vi "Recrystallise.vi"(8 "error in (no error)":errorcluster, 11 "XAOMsetting":refnum<vi>) -> (0 "error out":errorcluster)   [LabVIEW 2019]
uses:
  controls/xAOMSettings/XAOMsetting.xctl
  controls/GlobalExp.vi
  <vilib>/Utility/error.llb/Error Cluster From Error Code.vi
  <vilib>/rvi/errors/niLvFpgaAdjustHostInterfaceError.vi
  <vilib>/rvi/interface/nirviReadWriteControl/nirviReadWriteControl.xnode
  NiFpgaLv.dll
  <vilib>/rvi/interface/Simulation/niFpgaSimulationCallBeginRW.vi
  Global.lvlib
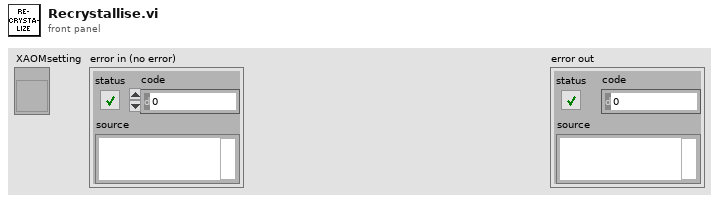
[diagram p1: front panel]
types:
  T1 = cluster{"HighPowerNum":dbl, "LowPowerNum":dbl, "PIDnum":dbl, "DeltaFreq":dbl, "BaseFreq":dbl, "AOMout":dbl, "ButtonSelected":enum16{"PID", "Low", "High"}, "AO3":bool}
  T2 = typedef "MasterExpControl.ctl" = cluster{"Main Steps":dbl, "Main Runs":dbl, "ExpStatus":enum16{"Innit", "Stop", "Idle", "MainRunning", "AuxRunning"}, "Main Current Step":dbl, "ExpNum":dbl, "NewData":bool, "date":string, "command":string, "Stop":bool, "Pause":bool, "Mathematica":string, "Main/Meta":bool, "UpdateMath":bool, "Camera":bool, "MetaExpOver":bool, "NextMetaExp":bool}
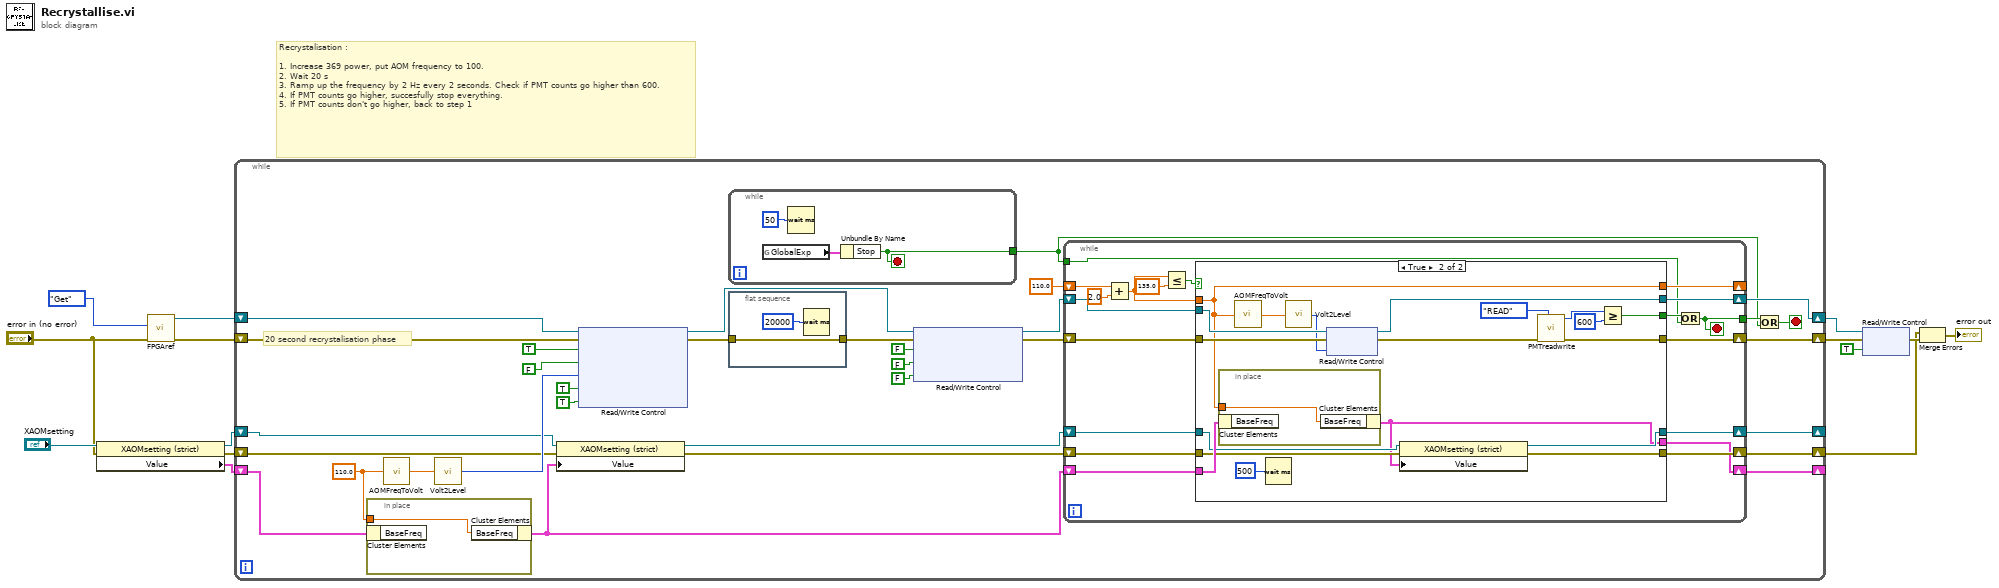
[diagram p0: block diagram]
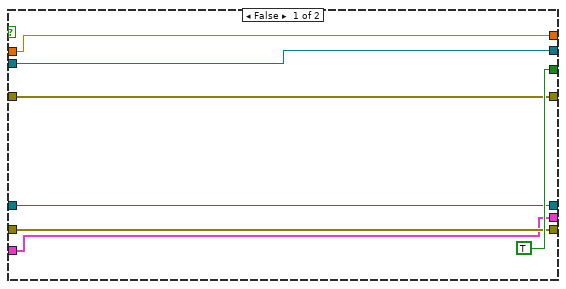
[diagram p2: hidden frame]
diagram:
  # "Recrystalisation :\n\n1. Increase 369 power, put AOM frequency to 100.\n2. Wait 20 s\n3. Ramp up the frequency by 2 Hz every 2 seconds. Check if PMT counts go higher than 600.\n4. If PMT counts go higher, succesfully stop everything.\n5. If PMT counts don't go higher, back to step 1"
  n1 = property class="XAOMsetting (strict)"(reference="XAOMsetting", error in="error in (no error)") -> (reference out=w9:refnum<vi>, error out=w7:errorcluster, "Value"=w8:T1)
  n2 = call "FPGAref.vi"("error in"="error in (no error)", "Enum"=enum16{"Set", "Get"}."Get") -> ("error out"=w5:errorcluster, "FPGA VI Reference Out 2"=w13:refnum<k20>)  [unwired: 4 in]
  n3 = while {
    shift-right: [w30] -> w12
    shift-left: w13 -> [w46]
    shift-right: [w22] -> _
    shift-left: w9 -> [w27]
    shift-right: [w20] -> _
    shift-left: w8 -> [w29]
    shift-right: [w21] -> w2
    shift-left: w7 -> [w26]
    shift-right: [w18] -> w4
    shift-left: w5 -> [w19]
    stop <- w17 stop-if-true
    w28 = 110.0 ("AOM freq")
    # "20 second recrystalisation phase"
    n4 = in-place {
      in-place-border: w28 -> [w50]
      n5 = in-place-cluster #1(w29) -> ()  [unwired: 1 out]
      n6 = in-place-cluster #1("BaseFreq"=w50) -> (w23:T1)
    }
    n7 = call "AOMFreqToVolt.vi"("AOM freq"=w28) -> ("AOM voltage"=w42:dbl)
    n8 = call "Volt2Level.vi"("voltage /V"=w42) -> ("level"=w43:i16)
    n9 = property class="XAOMsetting (strict)"(reference=w27, error in=w26, "Value"=w23) -> (reference out=w25:refnum<vi>, error out=w24:errorcluster)
    n10 = xnode "Read/Write Control"("FPGA VI Reference In"=w46, "error in"=w19, "AO4"=TRUE, "AO3"=FALSE, "AO3 off"=w43, "High power"=TRUE, "override noise eater?"=TRUE) -> ("FPGA VI Reference Out"=w40:refnum<k20>, "error out"=w41:errorcluster)
    n11 = while {
      tunnel: [w47] -> w15
      stop <- w47 stop-if-true
      n12 = global read "GlobalExp.vi" "GlobalExp"() -> (w49:T2)
      n13 = Wait (ms)(milliseconds to wait=u32 50) -> ()  [unwired: 1 out]
      n14 = Unbundle By Name(w49) -> ("Stop"=w47:bool)
    }
    n15 = flat-sequence {
      tunnel: [w97] -> w39
      tunnel: w41 -> [w97]
      frame #0 {
        n16 = Wait (ms)(milliseconds to wait=u32 20000) -> ()  [unwired: 1 out]
      }
    }
    n17 = xnode "Read/Write Control"("FPGA VI Reference In"=w40, "error in"=w39, "AO4"=FALSE, "High power"=FALSE, "override noise eater?"=FALSE) -> ("FPGA VI Reference Out"=w33:refnum<k20>, "error out"=w32:errorcluster)
    n18 = while {
      shift-right: [w61] -> w30
      shift-left: w33 -> [w67]
      shift-right: [w62] -> w18
      shift-left: w32 -> [w66]
      shift-right: [w60] -> _
      shift-left: 110.0 -> [w69]
      tunnel: [w52] -> w16
      shift-right: [w58] -> w22
      shift-left: w25 -> [w56]
      shift-right: [w57] -> w21
      shift-left: w24 -> [w55]
      shift-right: [w54] -> w20
      shift-left: w23 -> [w59]
      tunnel: w15 -> [w51]
      stop <- w52 stop-if-true
      n19 = Add(x=w69, y=2.0) -> (x+y=w64:dbl)
      n20 = Less Or Equal?(x=w64, y=135.0) -> (x <= y?=w65:bool)
      n21 = case shown="True" w65 {
        tunnel: w67 -> [w74 w94]
        tunnel: w66 -> [w75 w93]
        tunnel: w64 -> [w73 w84]
        tunnel: [TRUE w77] -> w53
        tunnel: [w75 w86] -> w62
        tunnel: [w74 w87] -> w61
        tunnel: [w73 w84] -> w60
        tunnel: w59 -> [w70 w85]
        tunnel: [w72 w83] -> w58
        tunnel: [w71 w82] -> w57
        tunnel: w56 -> [w72 w81]
        tunnel: w55 -> [w71 w80]
        tunnel: [w70 w79] -> w54
        frame False {
        }
        frame True {
          n22 = in-place {
            in-place-border: w84 -> [w96]
            n23 = in-place-cluster #2(w85) -> ()  [unwired: 1 out]
            n24 = in-place-cluster #2("BaseFreq"=w96) -> (w79:T1)
          }
          n25 = call "AOMFreqToVolt.vi"("AOM freq"=w84) -> ("AOM voltage"=w92:dbl)
          n26 = Wait (ms)(milliseconds to wait=u32 500) -> ()  [unwired: 1 out]
          n27 = call "Volt2Level.vi"("voltage /V"=w92) -> ("level"=w91:i16)
          n28 = xnode "Read/Write Control"("FPGA VI Reference In"=w94, "error in"=w93, "AO3 off"=w91) -> ("FPGA VI Reference Out"=w87:refnum<k20>, "error out"=w90:errorcluster)
          n29 = property class="XAOMsetting (strict)"(reference=w81, error in=w80, "Value"=w79) -> (reference out=w83:refnum<vi>, error out=w82:errorcluster)
          n30 = call "PMTreadwrite.vi"("Enum"=enum16{"READ", "WRITE"}."READ", "error in"=w90) -> ("error out"=w86:errorcluster, "Count Chart"=w89:u32)  [unwired: 8 in]
          n31 = Greater Or Equal?(x=w89, y=u32 600) -> (x >= y?=w77:bool)
        }
      }
      n32 = Or(x=w53, y=w51) -> (x .or. y?=w52:bool)
    }
    n33 = Or(x=w16, y=w15) -> (x .or. y?=w17:bool)
  }
  n34 = xnode "Read/Write Control"("FPGA VI Reference In"=w12, "error in"=w4, "AO3"=TRUE) -> ("error out"=w3:errorcluster)  [unwired: 1 out]
  n35 = Merge Errors(w2, w3) -> (→"error out":errorcluster)
